vi "ProdaNG.Tree.Release.Get.vi"(7 "TestStepsTree":refnum<vi>, 8 "error in (no error)":errorcluster, 9 "Release":bool) -> (0 "error out":errorcluster, 2 "Elements to release":T1[](array[typedef]))   [LabVIEW 2016]
uses:
  ProdaNG.Tree.Fglb.Data.ctl
  ProdaNG.Tree.Fglb.Element.ctl
  ProdaNG.Tree.Fglb.Action.ctl
  ProdaNG.Configurator.Glb.vi
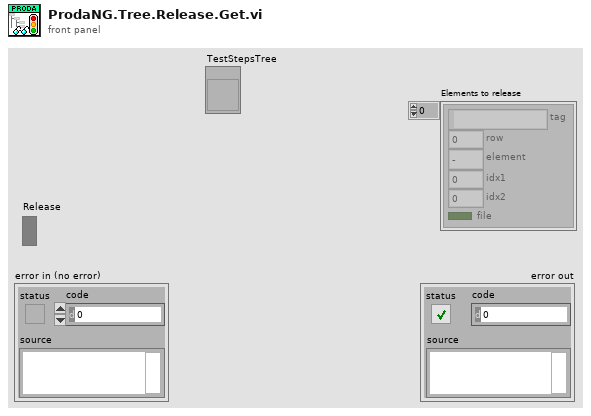
[diagram p1: front panel]
types:
  T1 = typedef "ProdaNG.Tree.Fglb.Data.ctl" = cluster{"tag":string, "row":i32, "element":T2, "idx1":i32, "idx2":i32, "file":bool}
  T2 = typedef "ProdaNG.Tree.Fglb.Element.ctl" = enum16{"-", "PP", "TS", "TP", "TV"}
  T3 = typedef "ProdaNG.Tree.Fglb.Action.ctl" = enum16{"init", "add", "get by row", "get by tag", "get by idx"}
  T4 = typedef "ProdaNG.TestStep.ctl" = cluster{"i_id":i32, "processStepId":i32, "testSequence":i32, "testOrder":i32, "mdReason":string, "mdUser":string, "mdTime":string, "description":string}
  T5 = typedef "ProdaNG.TestStepParam.ctl" = cluster{"i_id":i32, "testStepId":i32, "unitId":i32, "contentId":string, "previewId":string, "value":dbl, "valueText":string, "paramSequence":i32, "history":i32, "mdReason":string, "mdUser":string, "mdTime":string, "description":string}
  T6 = typedef "ProdaNG.TestValue.ctl" = cluster{"i_id":i32, "testStepId":i32, "releaseId":i32, "unitId":i32, "contentId":string, "previewId":string, "maximum":dbl, "minimum":dbl, "valueText":string, "testValueSequence":i32, "history":i32, "mdReason":string, "mdUser":string, "mdTime":string, "description":string}
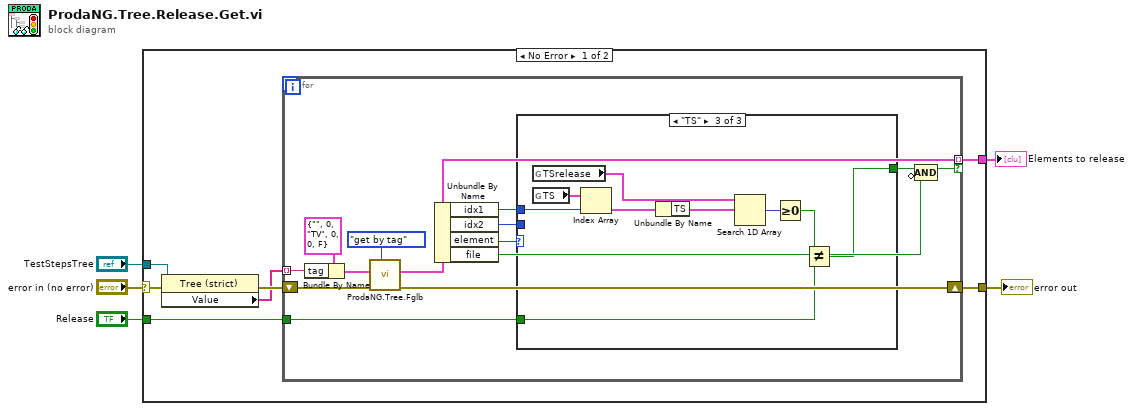
[diagram p0: block diagram]
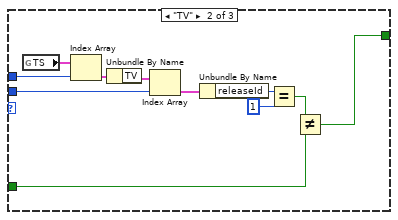
[diagram p3: hidden frame]
diagram:
  n1 = case shown="No Error" "error in (no error)" {
    selector: "error in (no error)" -> [w12 w47]
    tunnel: "TestStepsTree" -> [w9 _]
    tunnel: [w10 w47] -> w5
    tunnel: "Release" -> [w7 _]
    tunnel: [w6 _] -> w1
    frame No Error {
      n2 = property on="Property Node" class="Tree (strict)"(reference=w9, error in=w12) -> (error out=w11:errorcluster, "Value"=w8:string[])  [unwired: 1 out]
      n3 = for {
        tunnel: w8 -> [w23] mode=indexing
        shift-right: [w16] -> w10
        shift-left: w11 -> [w22]
        tunnel: w7 -> [w19]
        tunnel: [w18] -> w6 mode=indexing if=w14
        n4 = Bundle By Name(cluster=T1 {"tag"="", "row"=0, "element"=enum."TV", "idx1"=0, "idx2"=0, "file"=FALSE} ("entry in"), "tag"=w23) -> (w24:T1)
        n5 = call "ProdaNG.Tree.Fglb.vi"("Action (add)"=ProdaNG.Tree.Fglb.Action."get by tag", "error in"=w22, "entry in"=w24) -> ("error out"=w16:errorcluster, "found entry"=w18:T1)  [unwired: 6 in, 1 out]
        n6 = Unbundle By Name(w18) -> ("idx1"=w20:i32, "idx2"=w15:i32, "element"=w21:T2, "file"=w13:bool)
        n7 = case shown="\"TS\"" w21 {
          tunnel: w20 -> [_ w37 w45]
          tunnel: w19 -> [_ w31 w40]
          tunnel: [_ w30 w39] -> w17
          tunnel: w15 -> [_ w28 _]
          frame Default {
          }
          frame "TV" {
            n8 = global read "ProdaNG.Configurator.Glb.vi" "TS"() -> (w36:cluster{"TS":T4, "TP":T5[], "TV":T6[]}[])
            n9 = Index Array(array=w36, index=w37) -> (element=w35:cluster{"TS":T4, "TP":T5[], "TV":T6[]})
            n10 = Unbundle By Name(w35) -> ("TV"=w29:T6[])
            n11 = Index Array(array=w29, index=w28) -> (element=w27:T6)
            n12 = Unbundle By Name(w27) -> ("releaseId"=w34:i32)
            n13 = Equal?(x=w34, y=1) -> (x = y?=w32:bool)
            n14 = Not Equal?(x=w32, y=w31) -> (x != y?=w30:bool)
          }
          frame "TS" {
            n15 = global read "ProdaNG.Configurator.Glb.vi" "TSrelease"() -> (w43:T4[])
            n16 = global read "ProdaNG.Configurator.Glb.vi" "TS"() -> (w46:cluster{"TS":T4, "TP":T5[], "TV":T6[]}[])
            n17 = Index Array(array=w46, index=w45) -> (element=w44:cluster{"TS":T4, "TP":T5[], "TV":T6[]})
            n18 = Unbundle By Name(w44) -> ("TS"=w38:T4)
            n19 = Search 1D Array(1D array=w43, element=w38) -> (index of element=w42:i32)  [unwired: 1 in]
            n20 = Greater Or Equal To 0?(x=w42) -> (x >= 0?=w41:bool)
            n21 = Not Equal?(x=w41, y=w40) -> (x != y?=w39:bool)
          }
        }
        n22 = Compound Arithmetic op=AND(w17, invert w13) -> (w14:bool)
      }
    }
    frame Error {
    }
  }
  "error out" <- w5
  "Elements to release" <- w1
